vi "SACB FGV.vi"(6 "RH?":bool, 7 "Command":enum16{"Create", "Read", "Close"}(ring)=enum."Close", 8 "Error In":errorcluster) -> (0 "Error Out":errorcluster, 3 "Digital Inputs":T1)   [LabVIEW 2017]
uses:
  <vilib>/Modbus/master/Modbus Master.lvclass
  <vilib>/Modbus/master/Create Master Instance (TCP).vi
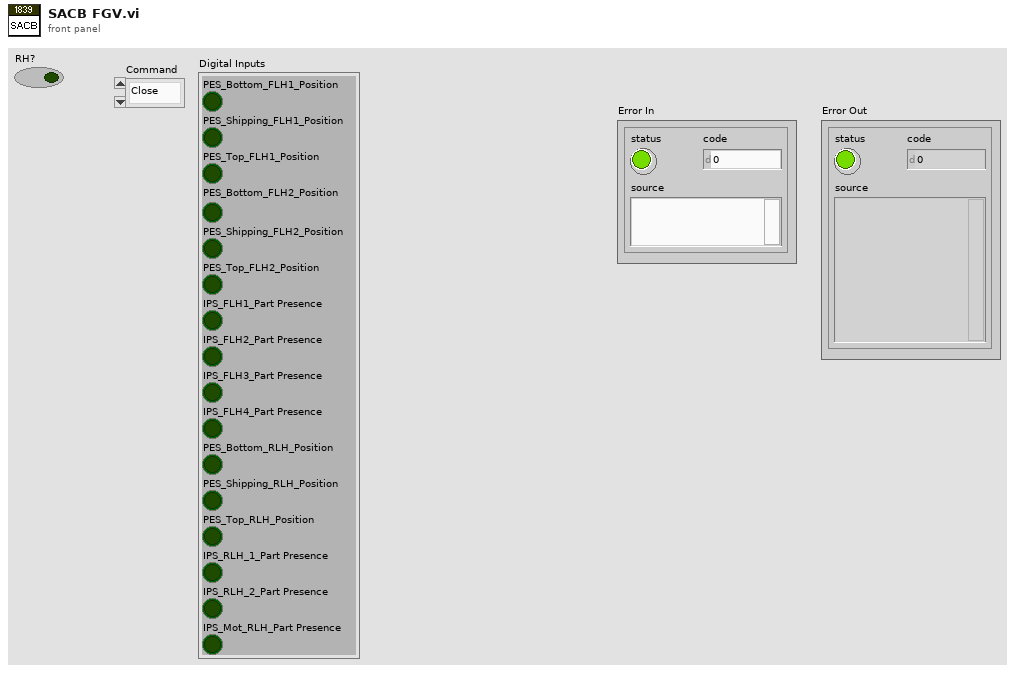
[diagram p1: front panel]
types:
  T1 = cluster{"PES_Bottom_FLH1_Position":bool, "PES_Shipping_FLH1_Position":bool, "PES_Top_FLH1_Position":bool, "PES_Bottom_FLH2_Position":bool, "PES_Shipping_FLH2_Position":bool, "PES_Top_FLH2_Position":bool, "IPS_FLH1_Part Presence":bool, "IPS_FLH2_Part Presence":bool, "IPS_FLH3_Part Presence":bool, "IPS_FLH4_Part Presence":bool, "PES_Bottom_RLH_Position":bool, "PES_Shipping_RLH_Position":bool, "PES_Top_RLH_Position":bool, "IPS_RLH_1_Part Presence":bool, "IPS_RLH_2_Part Presence":bool, "IPS_Mot_RLH_Part Presence":bool}
  T2 = cluster{"C0":bool, "C1":bool, "C2":bool, "C3":bool, "C4":bool, "C5":bool, "C6":bool, "C7":bool, "C7 2":bool, "C6 2":bool, "C5 2":bool, "C4 2":bool, "C3 2":bool, "C2 2":bool, "C1 2":bool, "C0 2":bool}
  T3 = cluster{"[0]":bool, "[1]":bool, "[2]":bool, "[3]":bool, "[4]":bool, "[5]":bool, "[6]":bool, "[7]":bool, "[8]":bool, "[9]":bool, "[10]":bool, "[11]":bool, "[12]":bool, "[13]":bool, "[14]":bool, "[15]":bool}
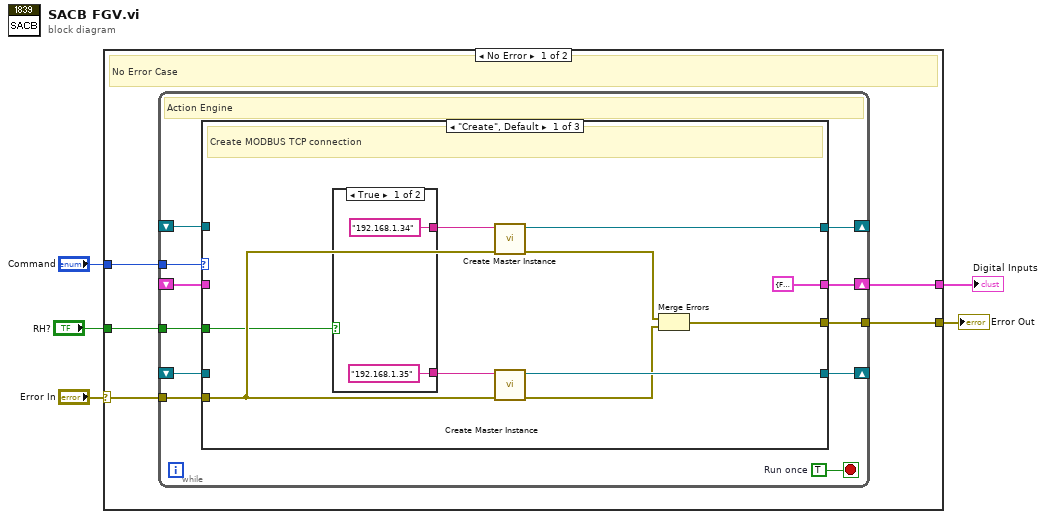
[diagram p0: block diagram]
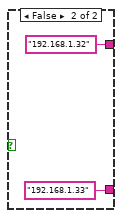
[diagram p2: hidden frame]
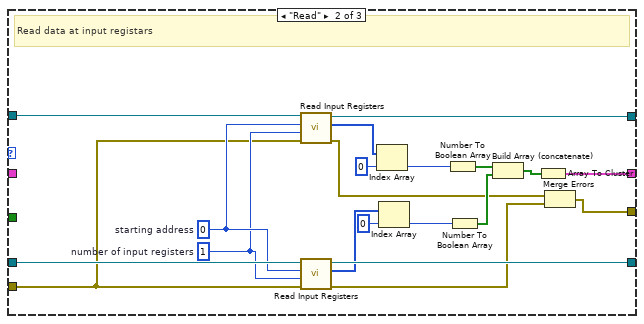
[diagram p3: hidden frame]
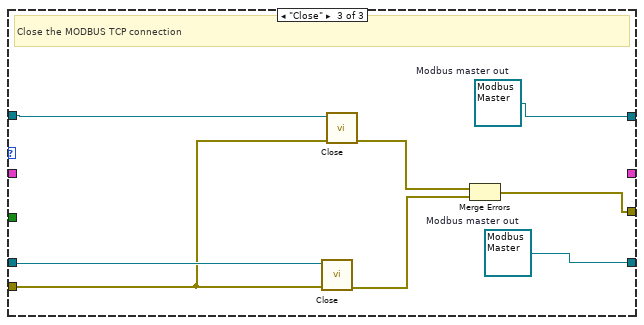
[diagram p4: hidden frame]
diagram:
  n1 = case shown="No Error" "Error In" {
    selector: "Error In" -> [w10 w64]
    tunnel: [w6 w64] -> w4
    tunnel: "Command" -> [w9 _]
    tunnel: [w8 _] -> w2
    tunnel: "RH?" -> [w7 _]
    frame No Error {
      # "No Error Case"
      n2 = while {
        tunnel: w9 -> [w20]
        shift-right: [w18] -> _
        shift-left: _ -> [w17]
        shift-right: [w16] -> w8
        shift-left: _ -> [w15]
        shift-right: [w14] -> _
        shift-left: _ -> [w13]
        tunnel: w10 -> [w21]
        tunnel: w7 -> [w12]
        tunnel: [w11] -> w6
        stop <- w19 stop-if-true
        w19 = TRUE  # Run once
        # "Action Engine"
        n3 = case shown="\"Create\", Default" w20 {
          tunnel: [w22 w36 w56] -> w11
          tunnel: w21 -> [w27 w39 w60]
          tunnel: [w30 w55 w62] -> w18
          tunnel: w17 -> [_ w54 w63]
          tunnel: [T2 {"C0"=FALSE, "C1"=FALSE, "C2"=FALSE, "C3"=FALSE, "C4"=FALSE, "C5"=FALSE, "C6"=FALSE, "C7"=FALSE, "C7 2"=FALSE, "C6 2"=FALSE, "C5 2"=FALSE, "C4 2"=FALSE, "C3 2"=FALSE, "C2 2"=FALSE, "C1 2"=FALSE, "C0 2"=FALSE} ("Digital Inputs 2") w40 _] -> w16
          tunnel: w15 -> [_ _ _]
          tunnel: [w29 w48 w59] -> w14
          tunnel: w13 -> [_ w46 w61]
          tunnel: w12 -> [w25 _ _]
          frame "Create", Default {
            # "Create MODBUS TCP connection"
            n4 = case shown="True" w25 {
              tunnel: ["192.168.1.35" ("address") "192.168.1.33" ("address")] -> w31
              tunnel: ["192.168.1.34" ("address") "192.168.1.32" ("address")] -> w28
              frame True {
              }
              frame False {
              }
            }
            n5 = call-poly <vilib>:"Create Master Instance.vi"("error in (no error)"=w27, "address"=w28) -> ("error out"=w24:errorcluster, "TCP master instance"=w29:refnum<class "Modbus Master.lvclass">)  [unwired: 8 in]
            n6 = call-poly <vilib>:"Create Master Instance.vi"("error in (no error)"=w27, "address"=w31) -> ("error out"=w23:errorcluster, "TCP master instance"=w30:refnum<class "Modbus Master.lvclass">)  [unwired: 8 in]
            n7 = Merge Errors(w24, w23) -> (w22:errorcluster)
          }
          frame "Read" {
            w44 = u16 1  # number of input registers
            w45 = u16 0  # starting address
            # "Read data at input registars"
            n8 = call-dynamic "Read Input Registers.vi"("error in (no error)"=w39, "number of input registers"=w44, "starting address"=w45, "Modbus master in"=w46) -> ("error out"=w37:errorcluster, "register values"=w47:u16[], "Modbus master out"=w48:refnum<class "Modbus Master.lvclass">)  [unwired: 5 in]
            n9 = call-dynamic "Read Input Registers.vi"("error in (no error)"=w39, "number of input registers"=w44, "starting address"=w45, "Modbus master in"=w54) -> ("error out"=w38:errorcluster, "register values"=w52:u16[], "Modbus master out"=w55:refnum<class "Modbus Master.lvclass">)  [unwired: 5 in]
            n10 = Index Array(array=w47, index=0) -> (element=w49:u16)
            n11 = Index Array "Index Array"(array=w52, index=0) -> (element=w53:u16)
            n12 = Number To Boolean Array(number=w49) -> (Boolean array=w43:bool[])
            n13 = Number To Boolean Array(number=w53) -> (Boolean array=w42:bool[])
            n14 = Build Array (concatenate)(w43, w42) -> (w41:bool[])
            n15 = Array To Cluster(array=w41) -> (cluster=w40:T3)
            n16 = Merge Errors(w37, w38) -> (w36:errorcluster)
          }
          frame "Close" {
            w59 = refnum<class "Modbus Master.lvclass"> refnum  # Modbus master out
            w62 = refnum<class "Modbus Master.lvclass"> refnum  # Modbus master out
            # "Close the MODBUS TCP connection"
            n17 = call-dynamic "Close.vi"("error in (no error)"=w60, "Modbus master in"=w63) -> ("error out"=w58:errorcluster)  [unwired: 9 in]
            n18 = call-dynamic "Close.vi"("error in (no error)"=w60, "Modbus master in"=w61) -> ("error out"=w57:errorcluster)  [unwired: 9 in]
            n19 = Merge Errors(w57, w58) -> (w56:errorcluster)
          }
        }
      }
    }
    frame Error {
      # "Error Handling Case"
    }
  }
  "Error Out" <- w4
  "Digital Inputs" <- w2
